vi "Read TDC Hits.vi"(7 "data value reference":T2, 8 "error in (no error)":errorcluster, 11 "TDCManager":T3) -> (0 "error out":errorcluster, 1 "Hits read":i32, 2 "Array":T1[](array[typedef]), 3 "TDCManager":T3, 6 "data value reference out":T2)   [LabVIEW 2016, in "HPTDC Driver Library.lvlib"]
uses:
  HPTDC Driver Library.lvlib
  Typedefs/TDCManager.ctl
  C:/Users/CRT Controller/CRTC Labview Application/Source/HPTDC Driver Library Folder/Library files/hptdc_net4_3.7.0_x64.dll
  hptdc_net4_3.7.0_x64.dll
  Typedefs/TDCHitArrayPointer.ctl
  Typedefs/TDCHit.ctl
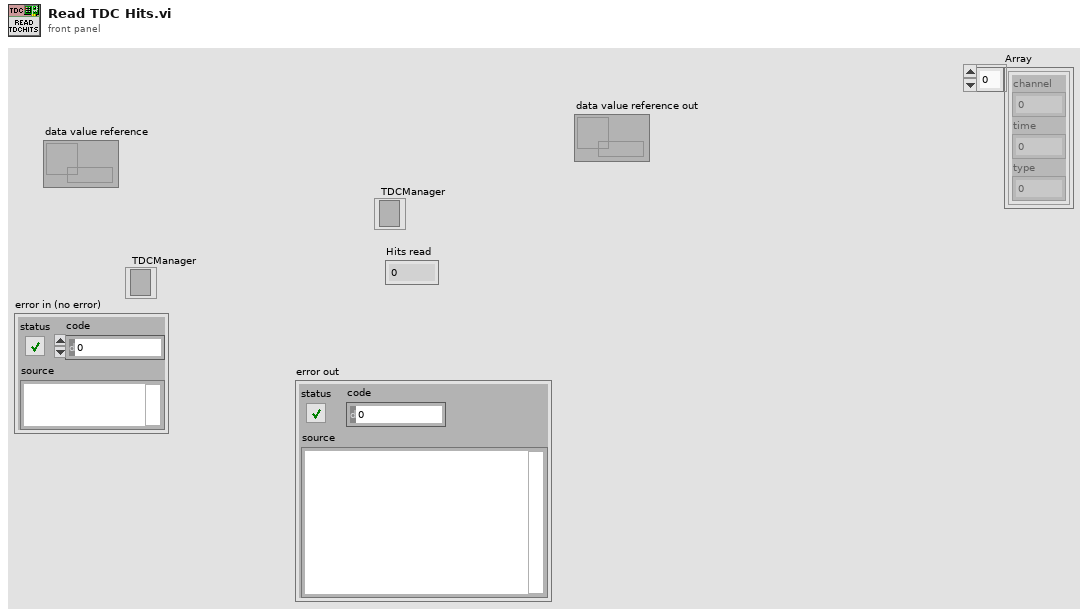
[diagram p1: front panel]
types:
  T1 = typedef "HPTDC Driver Library.lvlib/TDCHit.ctl" = cluster{"channel":u8, "time":u64, "type":u8}
  T2 = typedef "TDCHitArrayPointer.ctl" = refnum<data-value>
  T3 = typedef "HPTDC Driver Library.lvlib/TDCManager.ctl" = refnum<k24>
  T4 = typedef "Semaphore RefNum" = refnum<k1>
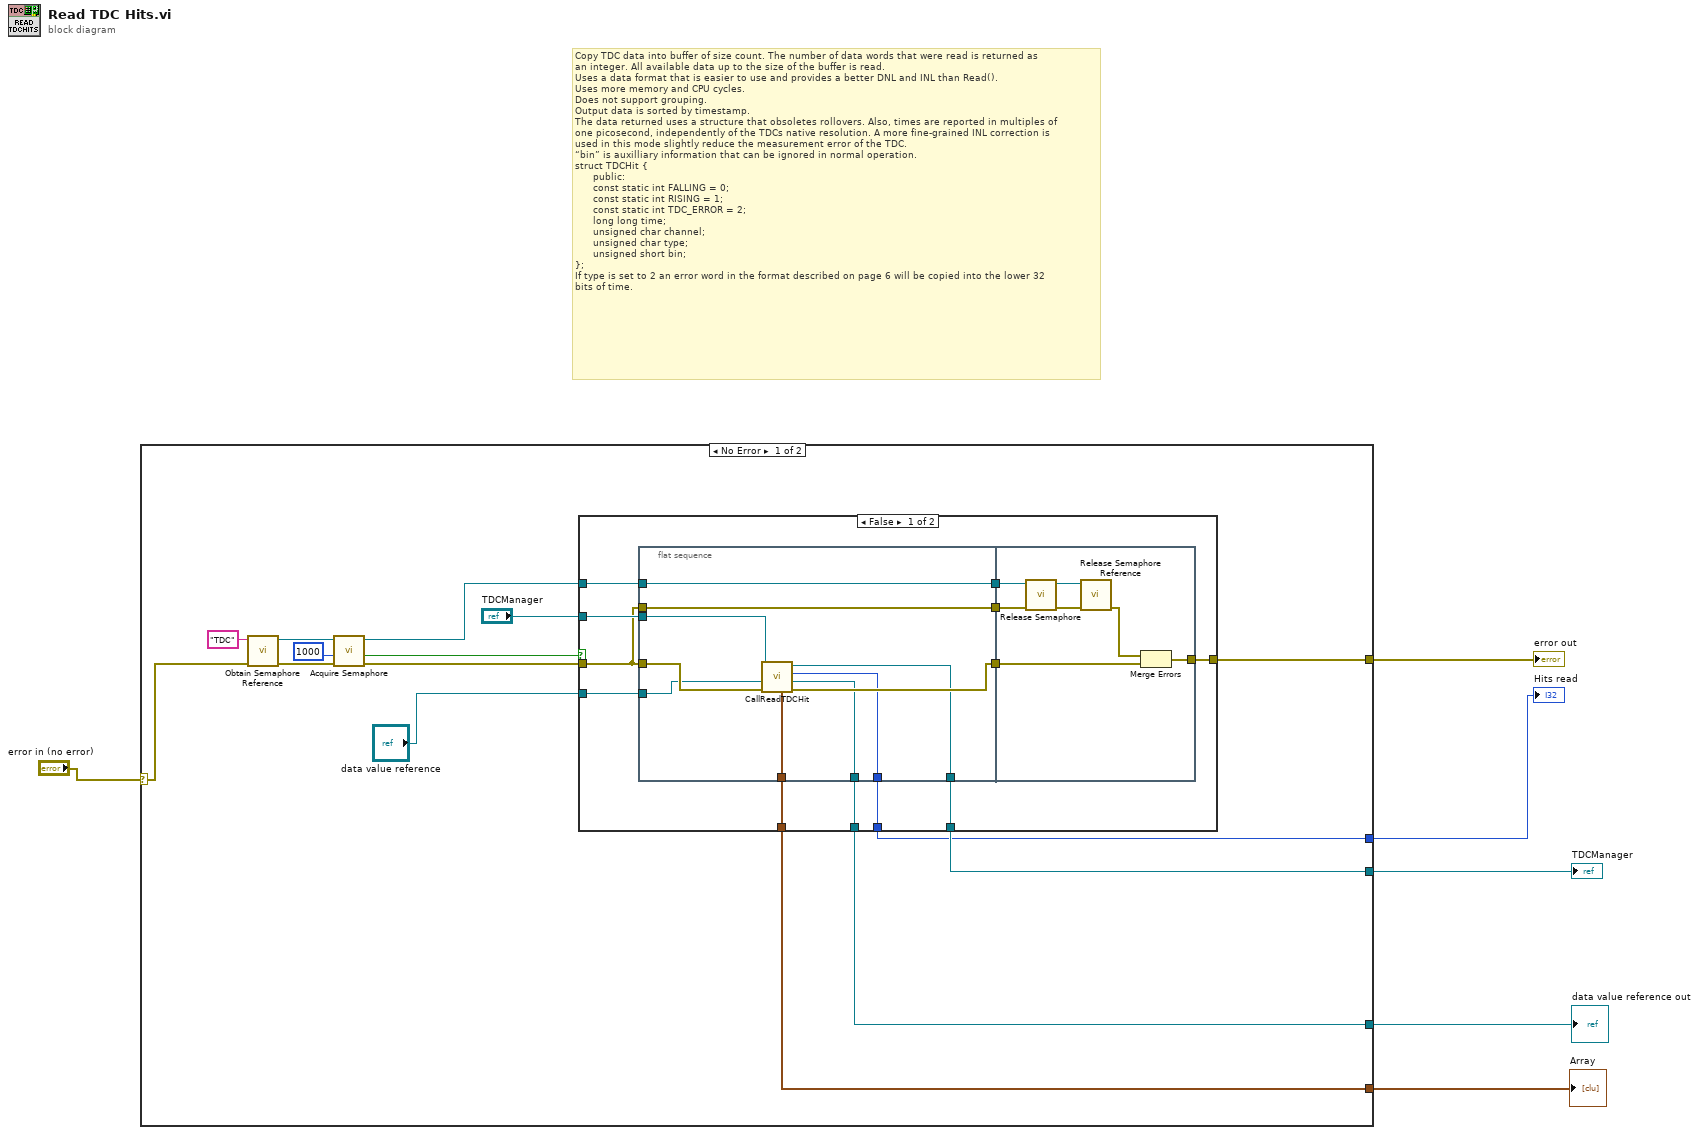
[diagram p0: block diagram]
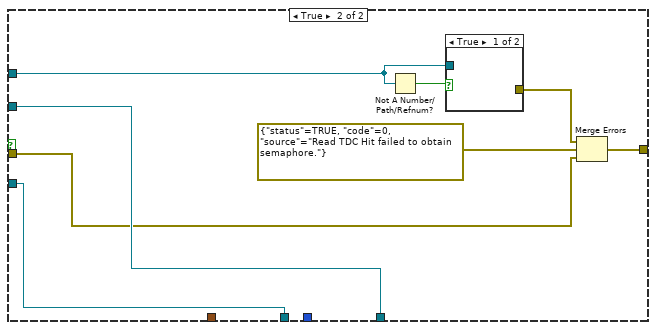
[diagram p2: hidden frame]
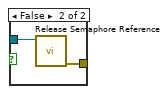
[diagram p3: hidden frame]
diagram:
  # "Copy TDC data into buffer of size count. The number of data words that were read is returned as\nan integer. All available data up to the size of the buffer is read.\nUses a data format that is easier to use and provides a better DNL and INL than Read().\nUses more memory and CPU cycles.\nDoes not support grouping.\nOutput data is sorted by timestamp.\nThe data returned uses a structure that obsoletes rollovers. Also, times are reported in multiples of\none picosecond, independently of the TDCs native resolution. A more fine-grained INL correction is\nused in this mode slightly reduce the measurement error of the TDC.\n“bin” is auxilliary information that can be ignored in normal operation.\nstruct TDCHit {\n      public:\n      const static int FALLING = 0;\n      const static int RISING = 1;\n      const static int TDC_ERROR = 2;\n      long long time;\n      unsigned char channel;\n      unsigned char type;\n      unsigned short bin;\n};\nIf type is set to 2 an error word in the format described on page 6 will be copied into the lower 32\nbits of time."
  n1 = case shown="No Error" "error in (no error)" {
    selector: "error in (no error)" -> [w7 w61]
    tunnel: [w13 _] -> w6
    tunnel: [w11 _] -> w5
    tunnel: [w10 _] -> w4
    tunnel: [w9 w61] -> w3
    tunnel: [w8 _] -> w2
    frame No Error {
      n2 = call <vilib>:"Obtain Semaphore Reference.vi"("error in (no error)"=w7, "name (unnamed)"="TDC") -> ("error out"=w19:errorcluster, "semaphore"=w20:T4)  [unwired: 3 in, 1 out]
      n3 = call <vilib>:"Acquire Semaphore.vi"("error in (no error)"=w19, "ms timeout (-1)"=1000, "semaphore"=w20) -> ("error out"=w16:errorcluster, "timed out"=w17:bool, "semaphore out"=w15:T4)  [unwired: 2 in]
      n4 = case shown="False" w17 {
        tunnel: "TDCManager" -> [w33 w58]
        tunnel: w16 -> [w30 w52]
        tunnel: w15 -> [w28 w54]
        tunnel: [w27 w58] -> w13
        tunnel: [w26 w56] -> w9
        tunnel: [w25 _] -> w10
        tunnel: "data value reference" -> [w23 w51]
        tunnel: [w24 w51] -> w11
        tunnel: [w22 _] -> w8
        frame False {
          n5 = flat-sequence {
            tunnel: w30 -> [w43]
            tunnel: w33 -> [w42]
            tunnel: [w41] -> w32
            tunnel: w30 -> [w40]
            tunnel: [w40] -> w31
            tunnel: [w39] -> w29
            tunnel: w28 -> [w39]
            tunnel: [w38] -> w27
            tunnel: [w37] -> w25
            tunnel: [w36] -> w24
            tunnel: w23 -> [w35]
            tunnel: [w34] -> w22
            tunnel: w32 -> [w44]
            tunnel: w31 -> [w48]
            tunnel: w29 -> [w46]
            tunnel: [w45] -> w26
            frame #0 {
              n6 = call "CallReadTDCHit.vi"("error in (no error)"=w43, "data value reference"=w35, ".NET Refnum in"=w42) -> ("error out"=w41:errorcluster, "data value reference out"=w36:T2, "# of hits read"=w37:i32, ".NET Refnum out"=w38:T3, "Array"=w34:T1[])  [unwired: 4 in]
            }
            frame #1 {
              n7 = call <vilib>:"Release Semaphore.vi"("error in (no error)"=w48, "semaphore"=w46) -> ("error out"=w49:errorcluster, "semaphore out"=w50:T4)  [unwired: 4 in]
              n8 = call <vilib>:"Release Semaphore Reference.vi"("error in (no error)"=w49, "semaphore"=w50) -> ("error out"=w47:errorcluster)  [unwired: 8 in, 1 out]
              n9 = Merge Errors(w47, w44) -> (w45:errorcluster)
            }
          }
        }
        frame True {
          n10 = Not A Number/Path/Refnum?(number/path/refnum=w54) -> (NaN/Path/Refnum?=w53:bool)
          n11 = case shown="True" w53 {
            tunnel: [_ w60] -> w55
            tunnel: w54 -> [_ w59]
            frame True {
            }
            frame False {
              n12 = call <vilib>:"Release Semaphore Reference.vi"("semaphore"=w59) -> ("error out"=w60:errorcluster)  [unwired: 9 in, 1 out]
            }
          }
          n13 = Merge Errors(w55, errorcluster {"status"=TRUE, "code"=0, "source"="Read TDC Hit failed to obtain semaphore."} ("error out"), w52) -> (w56:errorcluster)
        }
      }
    }
    frame Error {
    }
  }
  "TDCManager" <- w6
  "Hits read" <- w4
  "error out" <- w3
  "data value reference out" <- w5
  "Array" <- w2
